vi "PixieStartACQ.vi"(8 "error in (no error)":errorcluster, 10 "new run? (T)":bool=TRUE) -> (0 "error out":errorcluster)   [LabVIEW 2013]
doc: "Use this template to build a VI to use as a subVI."
uses:
  XIA/Pixie4/Drivers/Pixie4DLL.dll
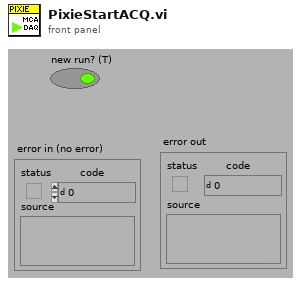
[diagram p1: front panel]
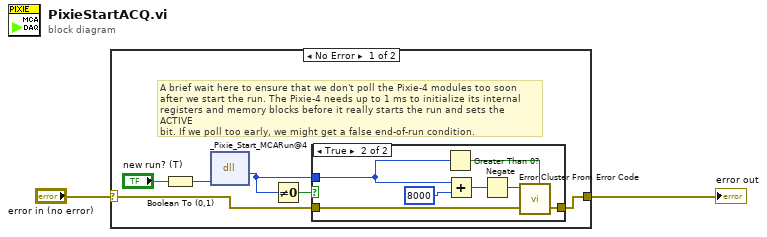
[diagram p0: block diagram]
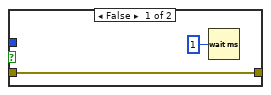
[diagram p2: hidden frame]
diagram:
  n1 = case shown="No Error" "error in (no error)" {
    selector: "error in (no error)" -> [w7 w18]
    tunnel: [w8 w18] -> w1
    frame No Error {
      # "A brief wait here to ensure that we don't poll the Pixie-4 modules too soon\nafter we start the run. The Pixie-4 needs up to 1 ms to initialize its internal\nregisters and memory blocks before it really starts the run and sets the ACTIVE\nbit. If we poll too early, we might get a false end-of-run condition."
      n2 = Boolean To (0,1)(Boolean="new run? (T)") -> (0, 1=w4:i16)
      n3 = dll-call lib="C:/XIA/Pixie4/Drivers/Pixie4DLL.dll" fn="_Pixie_Start_MCARun@4"("Mode"=w4) -> ("return type"=w5:i32)  [unwired: 4 in, 2 out]
      n4 = Not Equal To 0?(x=w5) -> (x != 0?=w6:bool)
      n5 = case shown="True" w6 {
        tunnel: w5 -> [_ w17]
        tunnel: [w10 w12] -> w8
        tunnel: w7 -> [w10 w11]
        frame False {
          n6 = Wait (ms)(milliseconds to wait=u32 1) -> ()  [unwired: 1 out]
        }
        frame True {
          n7 = Greater Than 0?(x=w17) -> (x > 0?=w14:bool)
          n8 = Add(x=w17, y=8000) -> (x+y=w15:i32)
          n9 = Negate(x=w15) -> (-x=w13:i32)
          n10 = call <vilib>:"Error Cluster From Error Code.vi"("is warning? (False)"=w14, "error in (no error)"=w11, "error code (0)"=w13) -> ("error out"=w12:errorcluster)  [unwired: 1 in, 5 out]
        }
      }
    }
    frame Error {
    }
  }
  "error out" <- w1
